vi "GPS_2.vi"() -> ()   [LabVIEW 2009]
uses:
  <vilib>/LabVIEW Targets/FPGA/cRIO/shared/nicrio_ModuleControls/nicrio_cRIO-9871_BaudRateEnum.ctl
  <vilib>/LabVIEW Targets/FPGA/cRIO/shared/nicrio_ModuleControls/nicrio_cRIO-9871_DataBitsEnum.ctl
  <vilib>/LabVIEW Targets/FPGA/cRIO/shared/nicrio_ModuleControls/nicrio_cRIO-9871_StopBitsEnum.ctl
  <vilib>/LabVIEW Targets/FPGA/cRIO/shared/nicrio_ModuleControls/nicrio_cRIO-9871_ParityEnum.ctl
  <vilib>/LabVIEW Targets/FPGA/cRIO/shared/nicrio_ModuleControls/nicrio_cRIO-9871_FlowControlEnum.ctl
  <vilib>/eio/EIOPropertyNode/EIOPropertyNode.xnode
  <vilib>/rvi/eio/nirviEIOPropertyImplementation/nirviEIOPropertyImplementation.xnode
  <vilib>/rvi/eio/common/nirviEmuTemplatePropertySet_errors.vi
  <vilib>/eio/EIOMethodNode/EIOMethodNode.xnode
  <vilib>/rvi/eio/nirviEIOMethodImplementation/nirviEIOMethodImplementation.xnode
  <vilib>/rvi/eio/common/nirviEmuTemplateMethod_errors.vi
  <vilib>/rvi/eio/common/nirviEmuClasses.ctl
  <vilib>/rvi/eio/common/nirviEmuTemplatePropertyGet_errors.vi
panel:
  out "GPS error out":errorcluster
  out "Output Started":bool
  out "Output Halted":bool
  out "Bytes at Port?":bool
  out "New GPS Data":bool
  out "GPS Data":u8[](array[numeric])
  out "Current Buffer":u8[](array[numeric])
  in  "GPS Read Timeout (us)":i32
  # "24"
  # "47"
  # "50"
  # "47"
  # "47"
  # "41"
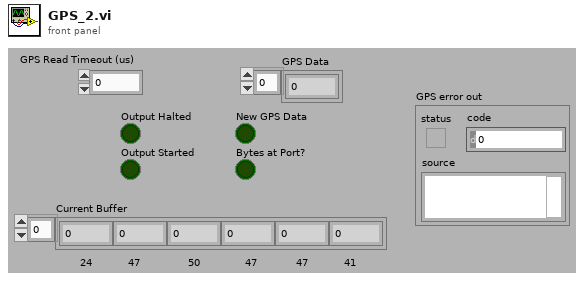
[diagram p1: front panel]
types:
  T1 = typedef "nicrio_cRIO-9871_FlowControlEnum.ctl" = enum8{"None", "Software (XON / XOFF)", "Hardware (RTS / CTS)"}
  T2 = typedef "nicrio_cRIO-9871_ParityEnum.ctl" = enum8{"None", "Odd", "Even", "Mark", "Space"}
  T3 = typedef "nicrio_cRIO-9871_StopBitsEnum.ctl" = enum8{"1", "1.5", "2"}
  T4 = typedef "nicrio_cRIO-9871_DataBitsEnum.ctl" = enum8{"5", "6", "7", "8"}
  T5 = typedef "nicrio_cRIO-9871_BaudRateEnum.ctl" = enum16{"75 bps", "110 bps", "134 bps", "150 bps", "300 bps", "600 bps", "1200 bps", "1800 bps", "2400 bps", "4800 bps", "7200 bps", "9600 bps", "14.4 kbps", "19.2 kbps", "28.8 kbps", "38.4 kbps", "57.6 kbps", "115.2 kbps", "230.4 kbps", "460.8 kbps", "921.6 kbps"}
  T6 = typedef "nirviEmuClasses.ctl" = enum16{"IO Read", "IO Write", "Method", "Property Read", "Property Write"}
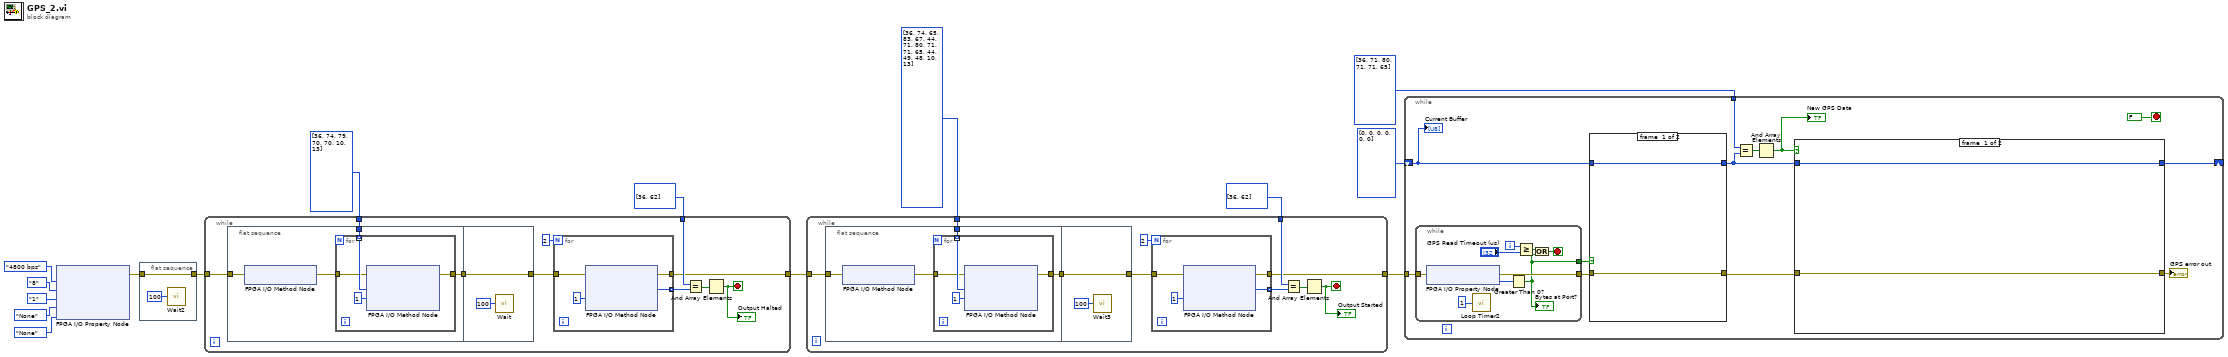
[diagram p0: block diagram]
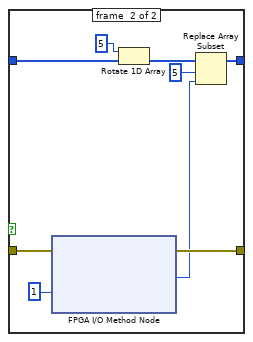
[diagram p2: hidden frame]
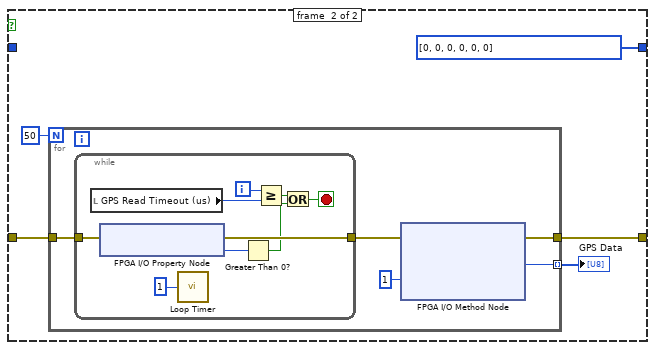
[diagram p3: hidden frame]
diagram:
  n1 = xnode "FPGA I/O Property Node"("Baud Rate"=nicrio_cRIO-9871_BaudRateEnum."4800 bps" ("Baud Rate 4"), "Data Bits"=nicrio_cRIO-9871_DataBitsEnum."8" ("Data Bits 4"), "Stop Bits"=nicrio_cRIO-9871_StopBitsEnum."1" ("Stop Bits 4"), "Parity"=nicrio_cRIO-9871_ParityEnum."None" ("Parity 4"), "Flow Control"=nicrio_cRIO-9871_FlowControlEnum."None" ("Flow Control 4")) -> ("error out"=w5:errorcluster)  [unwired: 2 in, 1 out]
  n2 = flat-sequence {
    tunnel: [w17] -> w6
    tunnel: w5 -> [w17]
    frame #0 {
      n3 = call "Wait2"("Count(mSec)"=u32 100) -> ()  [unwired: 1 out]
    }
  }
  n4 = while {
    tunnel: w6 -> [w26]
    tunnel: u8[] [36, 74, 79, 70, 70, 10, 13] -> [w25]
    tunnel: u8[] [36, 62] -> [w21]
    tunnel: [w18] -> w4
    stop <- w19 stop-if-true
    n5 = flat-sequence {
      tunnel: w26 -> [w30]
      tunnel: w25 -> [w29]
      tunnel: [w28] -> w24
      tunnel: w24 -> [w76]
      tunnel: [w76] -> w23
      frame #0 {
        n6 = xnode "FPGA I/O Method Node"("error in"=w30) -> ("error out"=w31:errorcluster)  [unwired: 1 in, 1 out]
        n7 = for {
          tunnel: w29 -> [w35] mode=indexing
          tunnel: w31 -> [w33]
          tunnel: [w32] -> w28
          n8 = xnode "FPGA I/O Method Node"("error in"=w33, "Data"=w35, "Timeout (ms)"=1) -> ("error out"=w32:errorcluster)  [unwired: 1 in, 2 out]
        }
      }
      frame #1 {
        n9 = call "Wait"("Count(mSec)"=u32 100) -> ()  [unwired: 1 out]
      }
    }
    n10 = for {
      N: 2 -> [_]
      tunnel: [w79] -> w22 mode=indexing
      tunnel: w23 -> [w78]
      tunnel: [w77] -> w18
      n11 = xnode "FPGA I/O Method Node"("error in"=w78, "Timeout (ms)"=1) -> ("error out"=w77:errorcluster, "Data"=w79:u8)  [unwired: 1 in, 2 out]
    }
    n12 = Equal?(x=w21, y=w22) -> (x = y?=w20:bool[])
    n13 = And Array Elements(Boolean array=w20) -> (logical AND=w19:bool)
    "Output Halted" <- w19
  }
  n14 = while {
    tunnel: w4 -> [w126]
    tunnel: u8[] [36, 74, 65, 83, 67, 44, 71, 80, 71, 71, 65, 44, 49, 48, 10, 13] -> [w125]
    tunnel: u8[] [36, 62] -> [w121]
    tunnel: [w118] -> w1
    stop <- w119 stop-if-true
    n15 = flat-sequence {
      tunnel: w126 -> [w128]
      tunnel: w125 -> [w130]
      tunnel: [w129] -> w124
      tunnel: w124 -> [w176]
      tunnel: [w176] -> w123
      frame #0 {
        n16 = xnode "FPGA I/O Method Node"("error in"=w128) -> ("error out"=w131:errorcluster)  [unwired: 1 in, 1 out]
        n17 = for {
          tunnel: w130 -> [w135] mode=indexing
          tunnel: w131 -> [w133]
          tunnel: [w132] -> w129
          n18 = xnode "FPGA I/O Method Node"("error in"=w133, "Data"=w135, "Timeout (ms)"=1) -> ("error out"=w132:errorcluster)  [unwired: 1 in, 2 out]
        }
      }
      frame #1 {
        n19 = call "Wait3"("Count(mSec)"=u32 100) -> ()  [unwired: 1 out]
      }
    }
    n20 = for {
      N: 2 -> [_]
      tunnel: [w179] -> w122 mode=indexing
      tunnel: w123 -> [w178]
      tunnel: [w177] -> w118
      n21 = xnode "FPGA I/O Method Node"("error in"=w178, "Timeout (ms)"=1) -> ("error out"=w177:errorcluster, "Data"=w179:u8)  [unwired: 1 in, 2 out]
    }
    n22 = Equal?(x=w121, y=w122) -> (x = y?=w120:bool[])
    n23 = And Array Elements(Boolean array=w120) -> (logical AND=w119:bool)
    "Output Started" <- w119
  }
  n24 = while {
    tunnel: w1 -> [w229]
    shift-right: [w220] -> _
    shift-left: u8[] [0, 0, 0, 0, 0, 0] -> [w223]
    tunnel: u8[] [36, 71, 80, 71, 71, 65] -> [w222]
    stop <- FALSE stop-if-true
    n25 = while {
      tunnel: w229 -> [w357]
      tunnel: [w356] -> w228
      tunnel: [w355] -> w221
      i -> [w362]
      stop <- w361 stop-if-true
      n26 = xnode "FPGA I/O Property Node"("error in"=w357) -> ("error out"=w356:errorcluster, "Bytes at Port"=w359:u8)  [unwired: 1 in, 1 out]
      n27 = call "Loop Timer2"("Count(uSec)"=u32 1) -> ()  [unwired: 1 out]
      n28 = Greater Than 0?(x=w359) -> (x > 0?=w355:bool)
      "Bytes at Port?" <- w355
      n29 = Greater Or Equal?(x=w362, y="GPS Read Timeout (us)") -> (x >= y?=w360:bool)
      n30 = Or(x=w360, y=w355) -> (x .or. y?=w361:bool)
    }
    n31 = case shown="True" w221 {
      tunnel: w228 -> [w231 w240]
      tunnel: [w231 w238] -> w226
      tunnel: w223 -> [w230 w234]
      tunnel: [w230 w235] -> w219
      frame #0 {
      }
      frame #1 {
        n32 = xnode "FPGA I/O Method Node"("error in"=w240, "Timeout (ms)"=1) -> ("error out"=w238:errorcluster, "Data"=w237:u8)  [unwired: 1 in, 2 out]
        n33 = Rotate 1D Array(1:w234, 2:5 ("n")) -> (0:w233:u8[])
        n34 = Replace Array Subset(array=w233, new element=w237, index=5) -> (w235:u8[])
      }
    }
    n35 = Equal?(x=w222, y=w219) -> (x = y?=w227:bool[])
    n36 = And Array Elements(Boolean array=w227) -> (logical AND=w225:bool)
    "New GPS Data" <- w225
    n37 = case shown="True" w225 {
      tunnel: w226 -> [w278 w283]
      tunnel: [w279 u8[] [0, 0, 0, 0, 0, 0]] -> w220
      tunnel: w219 -> [w279 _]
      tunnel: [w278 w280] -> w218
      frame #0 {
      }
      frame #1 {
        n38 = for {
          N: 50 -> [_]
          tunnel: w283 -> [w289]
          tunnel: [w286] -> w282 mode=indexing
          tunnel: [w285] -> w280
          n39 = while {
            tunnel: w289 -> [w293]
            tunnel: [w292] -> w288
            i -> [w297]
            stop <- w296 stop-if-true
            n40 = local read "GPS Read Timeout (us)"() -> (w290:i32)
            n41 = xnode "FPGA I/O Property Node"("error in"=w293) -> ("error out"=w292:errorcluster, "Bytes at Port"=w294:u8)  [unwired: 1 in, 1 out]
            n42 = call "Loop Timer"("Count(uSec)"=u32 1) -> ()  [unwired: 1 out]
            n43 = Greater Than 0?(x=w294) -> (x > 0?=w291:bool)
            n44 = Greater Or Equal?(x=w297, y=w290) -> (x >= y?=w295:bool)
            n45 = Or(x=w295, y=w291) -> (x .or. y?=w296:bool)
          }
          n46 = xnode "FPGA I/O Method Node"("error in"=w288, "Timeout (ms)"=1) -> ("error out"=w285:errorcluster, "Data"=w286:u8)  [unwired: 1 in, 2 out]
        }
        "GPS Data" <- w282
      }
    }
    "GPS error out" <- w218
    "Current Buffer" <- w223
  }
